vi "Init GPIO.vi"(7 "GPIO #":T3=-1, 8 "error in (no error)":errorcluster, 9 "GPIO Pull (None)":T2, 10 "GPIO Direction":T1, 11 "VisaSession in":refnum<class "VisaSession.lvclass">) -> (0 "error out":errorcluster, 2 "GPIO":refnum<class "GPIO.lvclass">, 3 "VisaSession out":refnum<class "VisaSession.lvclass">)   [LabVIEW 2020, in "CTI.lvlib" / "VisaSession.lvclass"]
uses:
  VisaSession.lvclass
  VisaSession.lvclass/VisaSession.ctl
  Session/Session.lvclass
  GPIO Number.ctl
  CTI.lvlib
  GPIO/GPIO.lvclass
  GPIO Pull.ctl
  GPIO Direction.ctl
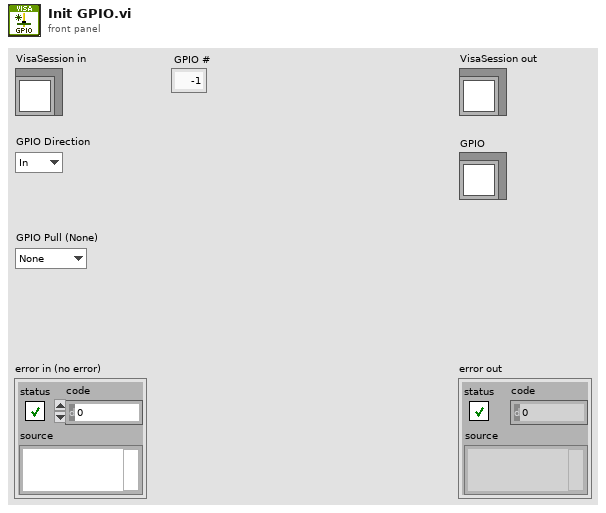
[diagram p1: front panel]
types:
  T1 = typedef "CTI.lvlib/GPIO Direction.ctl" = enum16{"In", "Out"}
  T2 = typedef "CTI.lvlib/GPIO Pull.ctl" = enum16{"None", "Up", "Down", "Both"}
  T3 = typedef "CTI.lvlib/GPIO Number.ctl" = i8
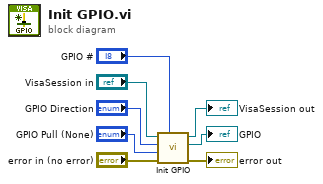
[diagram p0: block diagram]
diagram:
  n1 = call-parent "Init GPIO.vi"("GPIO #"="GPIO #", "error in (no error)"="error in (no error)", "GPIO Pull (None)"="GPIO Pull (None)", "GPIO Direction"="GPIO Direction", "Session in"="VisaSession in") -> ("error out"=→"error out":errorcluster, "GPIO"=→"GPIO":refnum<class "GPIO.lvclass">, "Session out"=→"VisaSession out":refnum<class "VisaSession.lvclass">)  [unwired: 4 in]
